vi "setActiveSheetIndex.vi"(8 "error in (no error)":errorcluster, 10 "ActiveSheetIndex":i32, 11 "workbook in":refnum<class "workbook.lvclass">) -> (0 "error out":errorcluster, 3 "workbook out":refnum<class "workbook.lvclass">)   [LabVIEW 2017, in "Excel_Specific.lvlib" / "workbook.lvclass"]
uses:
  workbook.lvclass
  workbook.lvclass/workbook.ctl
  C:/Users/Neo/Desktop/Dev_Tools_BR/LabVIEW_NPOI/src/lib/NPOI 2.1.1/NPOI.dll
  lib/NPOI 2.1.1/NPOI.dll
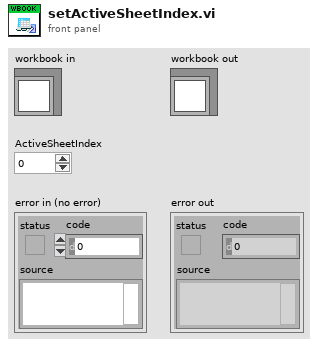
[diagram p1: front panel]
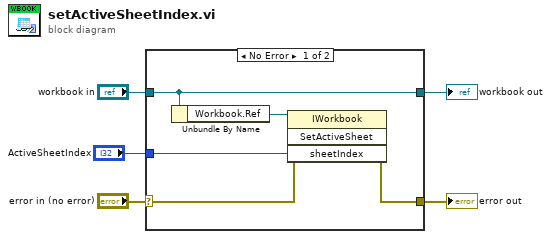
[diagram p0: block diagram]
diagram:
  n1 = case shown="No Error" "error in (no error)" {
    selector: "error in (no error)" -> [w8 w12]
    tunnel: [w7 w12] -> w4
    tunnel: [w10 w11] -> w2
    tunnel: "workbook in" -> [w10 w11]
    tunnel: "ActiveSheetIndex" -> [w6 _]
    frame No Error {
      n2 = Unbundle By Name(w10) -> ("Workbook.Ref"=w9:refnum<k24>)
      n3 = invoke class="IWorkbook" method="SetActiveSheet"(reference=w9, error in=w8, "sheetIndex"=w6) -> (error out=w7:errorcluster)  [unwired: 1 in, 3 out]
    }
    frame Error {
    }
  }
  "error out" <- w4
  "workbook out" <- w2
